vi "checkStateChange.vi"(4 "FieldRef":refnum<class "Field.lvclass">, 5 "distanceBehindBallToStealBall":dbl=400.0, 6 "Ball":refnum<class "Ball.lvclass">, 7 "State":T1=enum."KickToGoal", 8 "error in (no error)":errorcluster, 9 "enemyRobot":refnum<class "Robot.lvclass">, 10 "Robot in":refnum<class "Robot.lvclass">, 11 "ShootTactic in":refnum<class "ShootTactic.lvclass">) -> (0 "error out":errorcluster, 1 "pointBehindBall":dbl[](array[numeric]), 2 "canGoToKickToState?":bool, 3 "ShootTactic out":refnum<class "ShootTactic.lvclass">)   [LabVIEW 2023, in "ShootTactic.lvclass"]
uses:
  ShootTactic.lvclass
  Robot_class/Robot.lvclass
  C:/Users/ebert/Desktop/roboime/SSL_AI/Object_class/Object.lvclass
  Ball_class/Ball.lvclass
  States.ctl
  Field_class/Field.lvclass
  Object_class/Object.lvclass/Object.ctl
  Object_class/Read position(x,y).vi
  Utilities_class/Utilities.lvclass
  StealBallSkill_class/StealBallSkill.lvclass
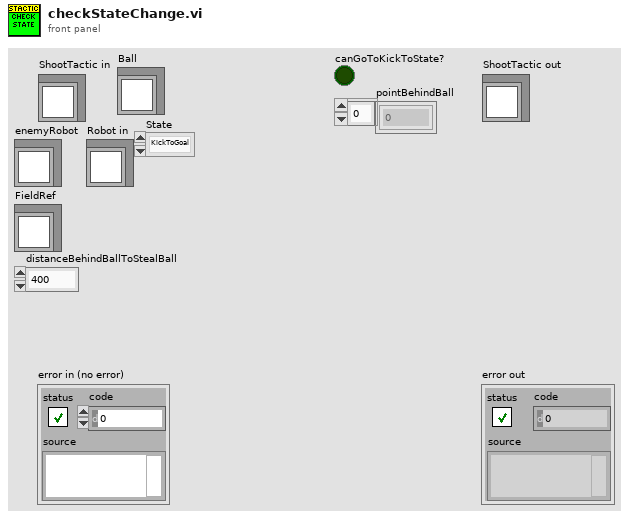
[diagram p1: front panel]
types:
  T1 = typedef "ShootTactic.lvclass/States.ctl" = enum16{"BallInGoalieArea", "Exit", "KickToGoal", "StealBall"}
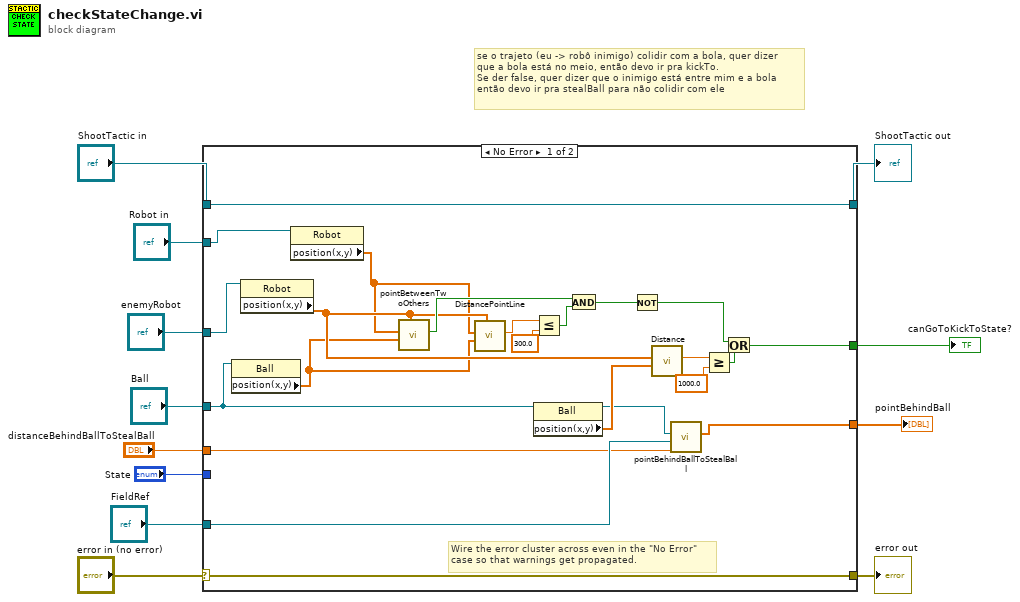
[diagram p0: block diagram]
diagram:
  # "se o trajeto (eu -> robô inimigo) colidir com a bola, quer dizer\nque a bola está no meio, então devo ir pra kickTo.\nSe der false, quer dizer que o inimigo está entre mim e a bola\nentão devo ir pra stealBall para não colidir com ele"
  n1 = case shown="No Error" "error in (no error)" {
    selector: "error in (no error)" -> [w34 w37]
    tunnel: [w34 w37] -> w11
    tunnel: [w35 w36] -> w9
    tunnel: "ShootTactic in" -> [w35 w36]
    tunnel: "enemyRobot" -> [w33 _]
    tunnel: "Ball" -> [w22 _]
    tunnel: "Robot in" -> [w23 _]
    tunnel: "State" -> [_ _]
    tunnel: [w32 _] -> w4
    tunnel: "FieldRef" -> [w27 _]
    tunnel: [w25 _] -> w2
    tunnel: "distanceBehindBallToStealBall" -> [w24 _]
    frame No Error {
      # "Wire the error cluster across even in the \"No Error\"\ncase so that warnings get propagated."
      n2 = property class="Ball"(reference=w22) -> ("position(x,y)"=w19:dbl[])  [unwired: 1 in, 2 out]
      n3 = property class="Robot"(reference=w33) -> ("position(x,y)"=w20:dbl[])  [unwired: 1 in, 2 out]
      n4 = property class="Robot"(reference=w23) -> ("position(x,y)"=w13:dbl[])  [unwired: 1 in, 2 out]
      n5 = call "pointBetweenTwoOthers.vi"("Query"=w20, "P2"=w19, "P1"=w13) -> ("queryBetweenP1P2"=w21:bool)  [unwired: 6 in, 2 out]
      n6 = call "DistancePointLine.vi"("Q"=w20, "P2"=w19, "P1"=w13) -> ("distance"=w18:dbl)  [unwired: 5 in, 3 out]
      n7 = Less Or Equal?(x=w18, y=300.0) -> (x <= y?=w17:bool)
      n8 = property class="Ball"(reference=w22) -> (reference out=w26:refnum<class "Ball.lvclass">, "position(x,y)"=w31:dbl[])  [unwired: 1 in, 1 out]
      n9 = And(x=w21, y=w17) -> (x .and. y?=w15:bool)
      n10 = Not(x=w15) -> (.not. x?=w14:bool)
      n11 = call "Distance.vi"("P1"=w31, "P2"=w20) -> ("Distance"=w30:dbl)  [unwired: 7 in, 2 out]
      n12 = call "pointBehindBallToStealBall.vi"("distanceBehindBallToStealBall"=w24, "Field"=w27, "Ball"=w26) -> ("pointBehindBall"=w25:dbl[])  [unwired: 8 in]
      n13 = Greater Or Equal?(x=w30, y=1000.0) -> (x >= y?=w28:bool)
      n14 = Or(x=w14, y=w28) -> (x .or. y?=w32:bool)
    }
    frame Error {
    }
  }
  "error out" <- w11
  "ShootTactic out" <- w9
  "canGoToKickToState?" <- w4
  "pointBehindBall" <- w2
